vi "Read.vi"(8 "error in (no error)":errorcluster, 11 "Bronkhorst Settings in":T1={"VISA resource name"="", "Simulated?"=FALSE, "Smoothing Steps"=1} {"Smoothing Steps" min=1 step=1}) -> (0 "error out":errorcluster, 1 "Connection Error":bool, 2 "flow":dbl, 3 "Bronkhorst Settings out":T1={"VISA resource name"="", "Simulated?"=FALSE, "Smoothing Steps"=1} {"Smoothing Steps" min=1 step=1})   [LabVIEW 2018, in "Bronkhorst M14 Flow Meter.lvlib"]
uses:
  Bronkhorst M14 Flow Meter.lvlib
  Settings Cluster.ctl
  <userlib>/_OpenG.lib/numeric/numeric.llb/Random Number Within Range - DBL__ogtk.vi
  <vilib>/regexp/Match Regular Expression.xnode
  <vilib>/ptbypt/NI_PtbyPt.lvlib
panel:
  out "whole match":string
  out "x/y":dbl
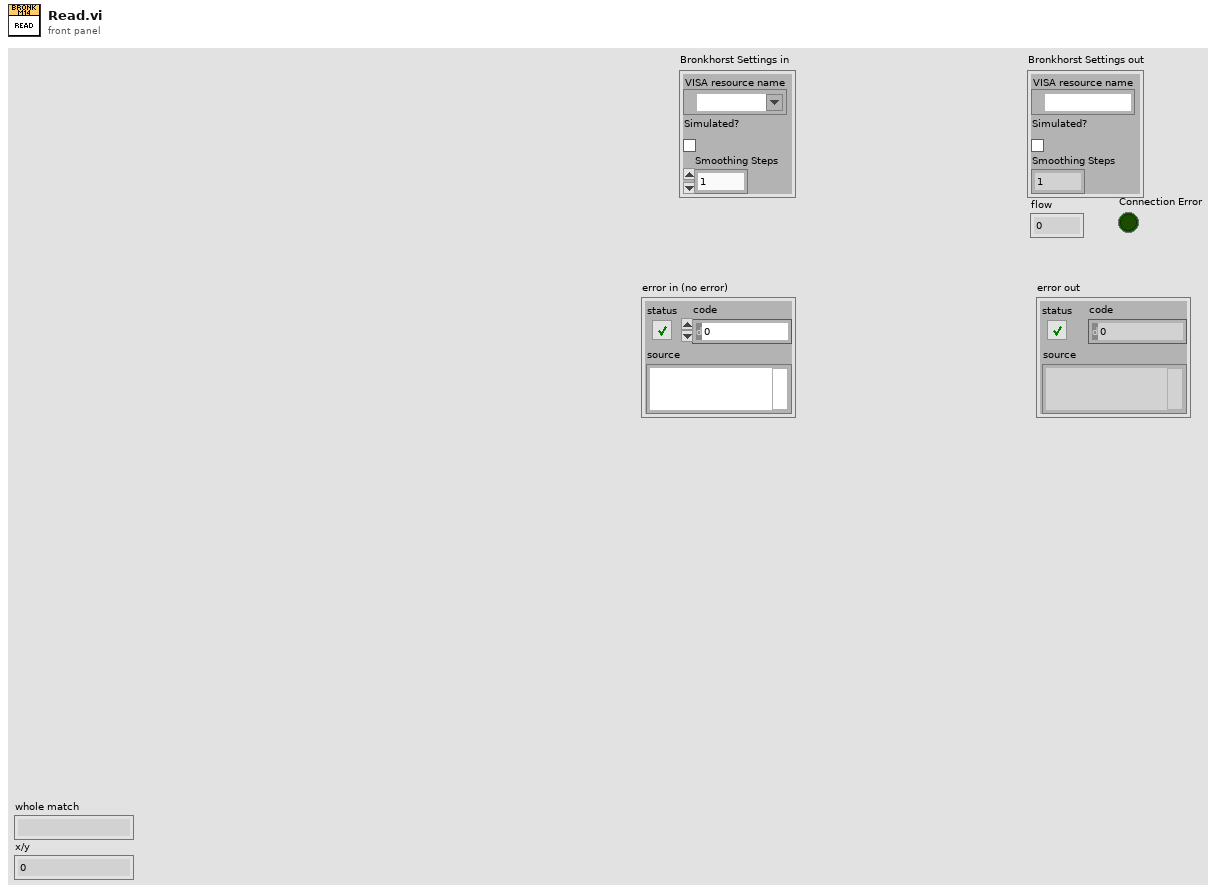
[diagram p1: front panel]
types:
  T1 = typedef "Bronkhorst M14 Flow Meter.lvlib/Settings Cluster.ctl" = cluster{"VISA resource name":refnum<visa-resource-name>, "Simulated?":bool, "Smoothing Steps":i32}
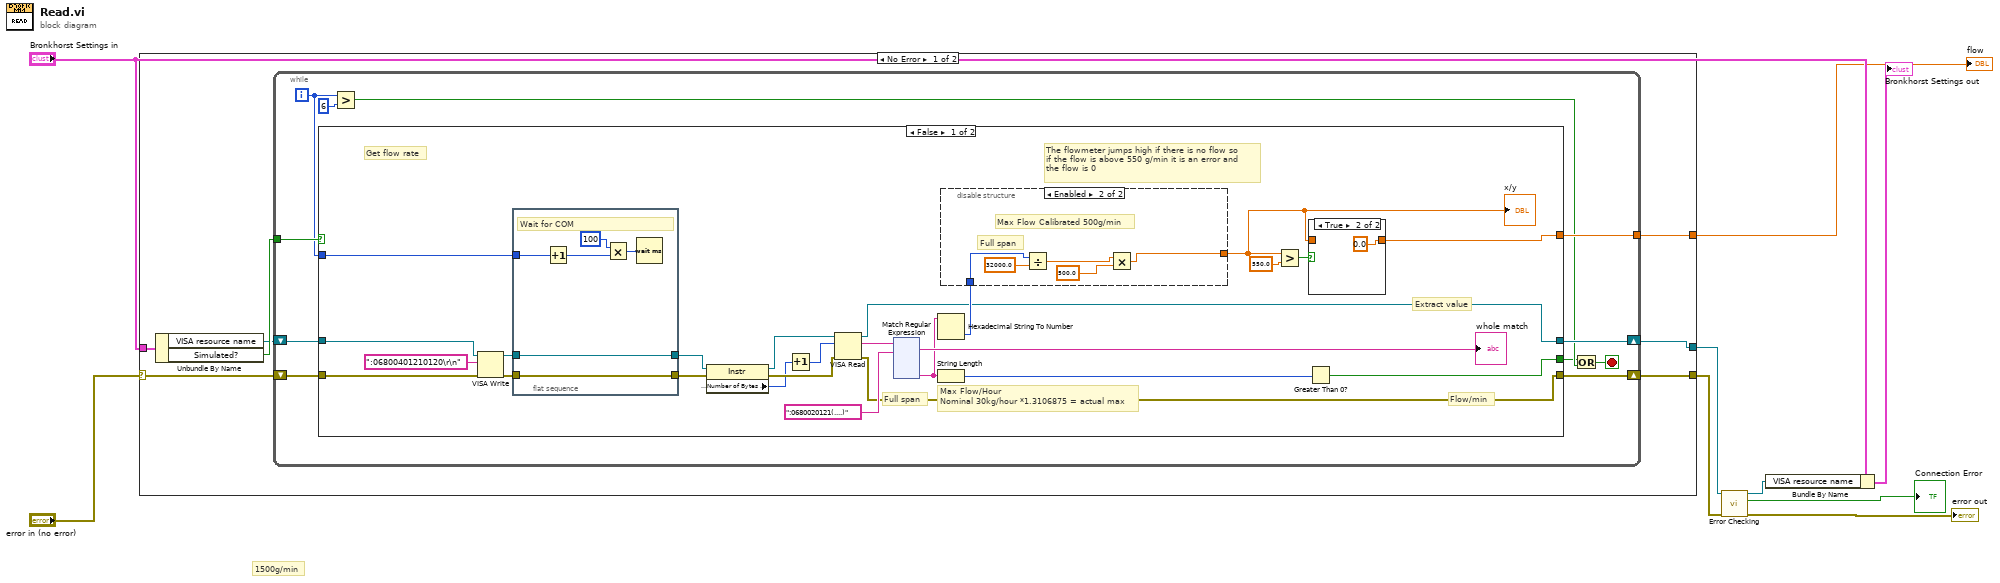
[diagram p0: block diagram]
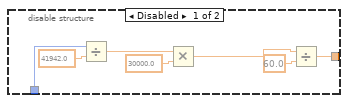
[diagram p2: hidden frame]
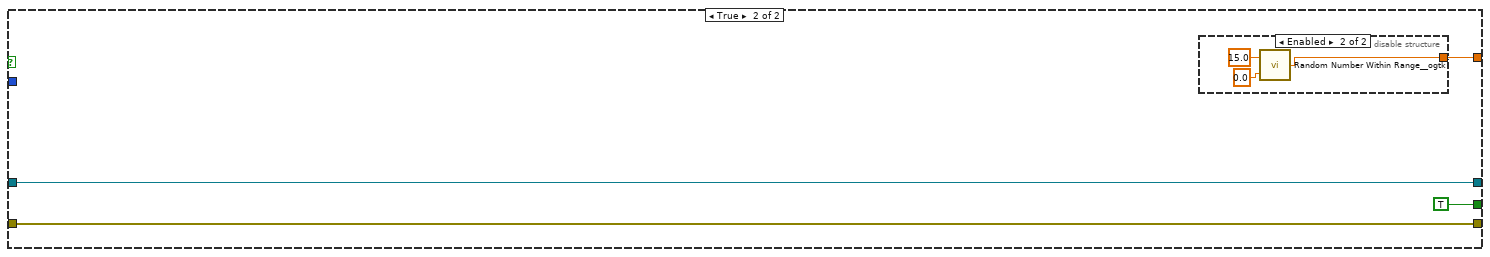
[diagram p4: hidden frame]
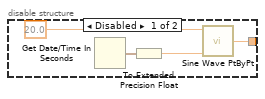
[diagram p5: hidden frame]
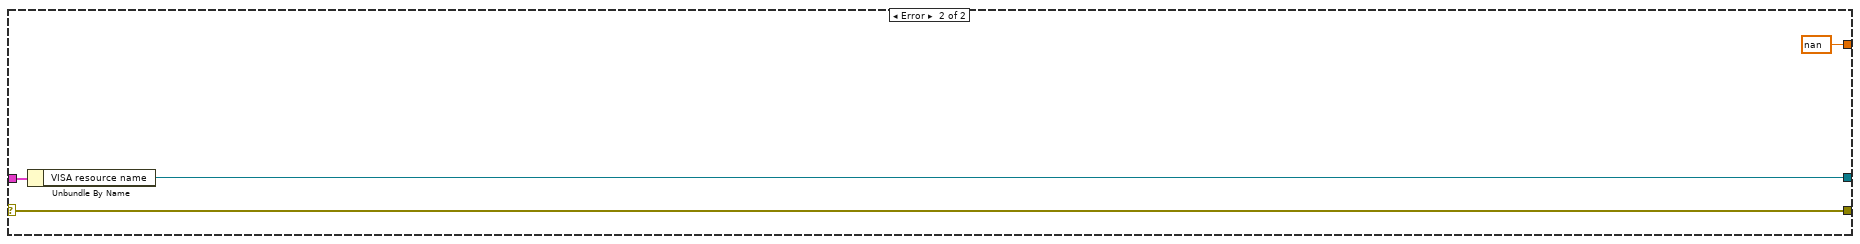
[diagram p6: hidden frame]
diagram:
  # "1500g/min"
  n1 = case shown="No Error" "error in (no error)" {
    selector: "error in (no error)" -> [w15 w203]
    tunnel: [w14 w203] -> w7
    tunnel: "Bronkhorst Settings in" -> [w12 w201]
    tunnel: [w13 nan ("sine wave")] -> w4
    tunnel: [w10 w200] -> w9
    frame No Error {
      n2 = Unbundle By Name(w12) -> ("VISA resource name"=w11:refnum<visa-resource-name>, "Simulated?"=w16:bool)
      n3 = while {
        tunnel: w16 -> [w27]
        tunnel: [w24] -> w13
        shift-right: [w25] -> w14
        shift-left: w15 -> [w26]
        shift-right: [w22] -> w10
        shift-left: w11 -> [w23]
        i -> [w18]
        stop <- w17 stop-if-true
        n4 = case shown="False" w27 {
          tunnel: [w32 w192] -> w25
          tunnel: w26 -> [w37 w192]
          tunnel: [w41 w189] -> w24
          tunnel: [w33 w191] -> w22
          tunnel: w23 -> [w38 w191]
          tunnel: [w28 TRUE] -> w19
          tunnel: w18 -> [w30 _]
          frame False {
            # "Flow/min"
            # "Max Flow/Hour\nNominal 30kg/hour *1.3106875 = actual max"
            # "Full span"
            # "Extract value"
            # "Get flow rate"
            # "The flowmeter jumps high if there is no flow so \nif the flow is above 550 g/min it is an error and \nthe flow is 0"
            n5 = VISA Write(VISA resource name=w38, write buffer=":06800401210120\r\n" ("Command"), error in (no error)=w37) -> (VISA resource name out=w49:refnum<visa-resource-name>, error out=w47:errorcluster)  [unwired: 1 out]
            n6 = flat-sequence {
              tunnel: [w188] -> w48
              tunnel: w49 -> [w188]
              tunnel: [w187] -> w46
              tunnel: w47 -> [w187]
              tunnel: w30 -> [w184]
              frame #0 {
                # "Wait for COM"
                n7 = Increment(x=w184) -> (x+1=w183:i32)
                n8 = Multiply(x=u32 100 ("milliseconds to wait"), y=w183) -> (x*y=w185:u32)
                n9 = Wait (ms)(milliseconds to wait=w185) -> ()  [unwired: 1 out]
              }
            }
            n10 = property class="Instr"(reference=w48, error in=w46) -> (reference out=w51:refnum<visa-resource-name>, error out=w50:errorcluster, "Serial Settings:Number of Bytes at Serial Port"=w35:u32)
            n11 = Increment(x=w35) -> (x+1=w34:u32)
            n12 = VISA Read(VISA resource name=w51, byte count=w34, error in (no error)=w50) -> (VISA resource name out=w33:refnum<visa-resource-name>, read buffer=w36:string, error out=w32:errorcluster)  [unwired: 1 out]
            n13 = xnode "Match Regular Expression"("input string"=w36, "regular expression"=":0680020121(....)" ("Regular Expression for Extracting Weight")) -> ("whole match"=→"whole match":string, "submatch 1"=w31:string)  [unwired: 4 in, 4 out]
            n14 = Hexadecimal String To Number(string=w31) -> (number=w39:u32)  [unwired: 2 in, 1 out]
            n15 = String Length(string=w31) -> (length=w29:i32)
            n16 = disable-structure shown="Enabled" {
              disable-tunnel: [w55 w60] -> w42
              disable-tunnel: w39 -> [w54 w64]
              frame Disabled {
                n17 = Divide(x=w54, y=41942.0) -> (x/y=w56:dbl)
                n18 = Multiply(x=w56, y=30000.0) -> (x*y=w53:dbl)
                n19 = Divide(x=w53, y=60.0) -> (x/y=w55:dbl)
              }
              frame Enabled {
                # "Full span"
                # "Max Flow Calibrated 500g/min"
                n20 = Divide(x=w64, y=32000.0) -> (x/y=w62:dbl)
                n21 = Multiply(x=w62, y=500.0) -> (x*y=w60:dbl)
              }
            }
            "x/y" <- w42
            n22 = Greater?(x=w42, y=550.0) -> (0:w43:bool)
            n23 = Greater Than 0?(x=w29) -> (x > 0?=w28:bool)
            n24 = case shown="True" w43 {
              tunnel: [w65 0.0] -> w41
              tunnel: w42 -> [w65 _]
              frame False {
              }
              frame True {
              }
            }
          }
          frame True {
            n25 = disable-structure shown="Enabled" {
              disable-tunnel: [w193 w197] -> w189
              frame Disabled {
                n26 = Get Date/Time In Seconds() -> (seconds since 1Jan1904=w196:timestamp)
                n27 = To Extended Precision Float(1:w196) -> (0:w195:ext)
                n28 = call <vilib>:"Sine Wave PtByPt.vi"("time"=w195, "amplitude"=20.0) -> ("sine wave"=w193:dbl)  [unwired: 2 in]
              }
              frame Enabled {
                n29 = call-poly <userlib>:"Random Number Within Range__ogtk.vi"("High"=15.0, "Low"=0.0) -> ("Random Number"=w197:dbl)  [unwired: 3 in]
              }
            }
          }
        }
        n30 = Greater?(x=w18, y=6) -> (0:w20:bool)
        n31 = Or(x=w19, y=w20) -> (x .or. y?=w17:bool)
      }
    }
    frame Error {
      n32 = Unbundle By Name(w201) -> ("VISA resource name"=w200:refnum<visa-resource-name>)
    }
  }
  "flow" <- w4
  n33 = call "Error Checking.vi"("error in (no error)"=w7, "VISA resource name"=w9) -> ("error out"=→"error out":errorcluster, "Connection Error"=→"Connection Error":bool, "VISA resource name"=w8:refnum<visa-resource-name>)  [unwired: 7 in]
  n34 = Bundle By Name(cluster="Bronkhorst Settings in", "VISA resource name"=w8) -> (→"Bronkhorst Settings out":T1)
